vi "2025_day2 - Validate Number.vi"(2 "Number to test In":u64) -> (4 "Reptetive Pattern Found? (Task 2)":bool, 7 "Number to test Out":u64, 8 "Reptetive Pattern Found? (Task 1)":bool)   [LabVIEW 2025]
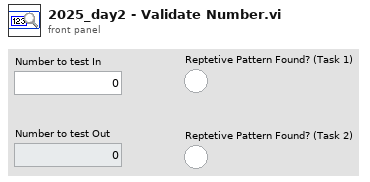
[diagram p1: front panel]
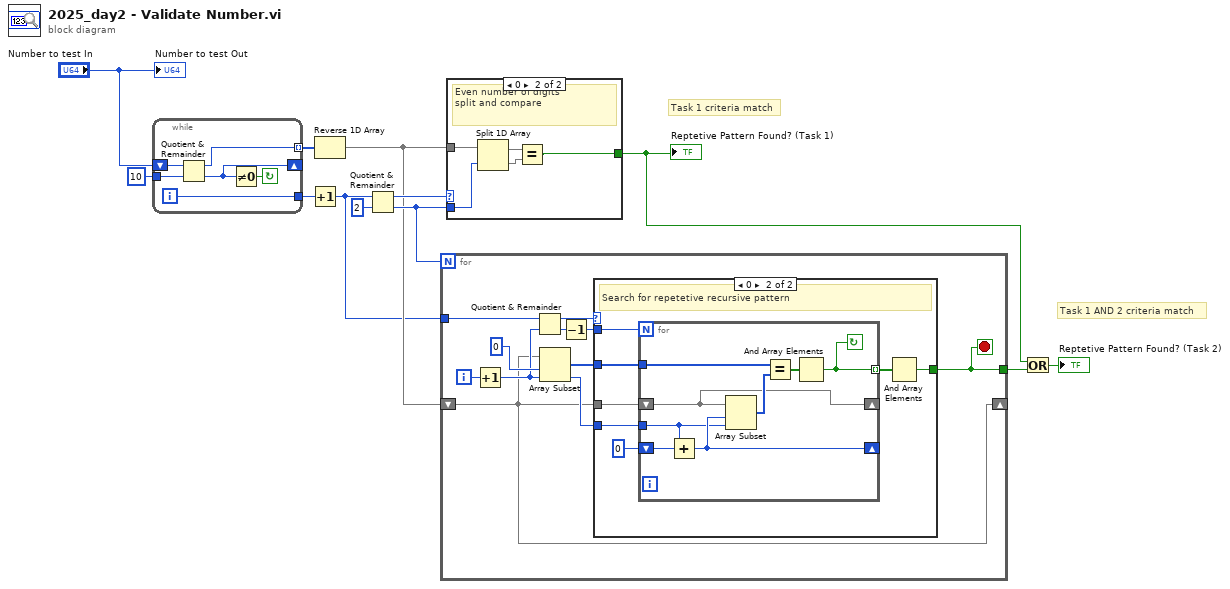
[diagram p0: block diagram]
diagram:
  # "Task 1 AND 2 criteria match"
  # "Task 1 criteria match"
  n1 = while {
    shift-right: [w14] -> _
    shift-left: "Number to test In" -> [w18]
    tunnel: 10 -> [w17]
    tunnel: [w16] -> w11 mode=indexing
    tunnel: [w13] -> w10
    i -> [w13]
    stop <- w15 continue-if-true
    n2 = Quotient & Remainder(x=w18, y=w17) -> (x-y*floor(x/y)=w16:u64, floor(x/y)=w14:u64)
    n3 = Not Equal To 0?(x=w14) -> (x != 0?=w15:bool)
  }
  n4 = Increment(x=w10) -> (x+1=w4:i32)
  n5 = Reverse 1D Array(array=w11) -> (reversed array=w5:u64[])
  n6 = Quotient & Remainder(x=w4, y=2) -> (x-y*floor(x/y)=w8:i32, floor(x/y)=w6:i32)
  n7 = for {
    N: w6 -> [_]
    shift-right: [w21] -> _
    shift-left: w5 -> [w21]
    tunnel: w4 -> [w26]
    tunnel: [w20] -> w3
    i -> [w28]
    stop <- w20 stop-if-true
    n8 = Increment(x=w28) -> (x+1=w23:i32)
    n9 = Quotient & Remainder(x=w26, y=w23) -> (x-y*floor(x/y)=w25:i32, floor(x/y)=w24:i32)
    n10 = Array Subset(array=w21, index=0, length=w23) -> (w22:u64[])
    n11 = Decrement(x=w24) -> (x-1=w19:i32)
    n12 = case shown="0" w25 {
      tunnel: w21 -> [_ w35]
      tunnel: w19 -> [_ w34]
      tunnel: w23 -> [_ w32]
      tunnel: w22 -> [_ w31]
      tunnel: [_ w29] -> w20
      frame Default {
        # "No Match possible"
      }
      frame 0 {
        # "Search for repetetive recursive pattern"
        n13 = for {
          N: w34 -> [_]
          shift-right: [w42] -> _
          shift-left: 0 ("index") -> [w43]
          tunnel: w32 -> [w41]
          tunnel: w31 -> [w40]
          tunnel: [w36] -> w30 mode=indexing
          shift-right: [w37] -> _
          shift-left: w35 -> [w37]
          stop <- w36 continue-if-true
          n14 = Add(x=w43, y=w41) -> (x+y=w42:i32)
          n15 = Array Subset(array=w37, index=w42, length=w41) -> (w39:u64[])
          n16 = Equal?(x=w40, y=w39) -> (x = y?=w38:bool[])
          n17 = And Array Elements(Boolean array=w38) -> (logical AND=w36:bool)
        }
        n18 = And Array Elements(Boolean array=w30) -> (logical AND=w29:bool)
      }
    }
  }
  n19 = case shown="0" w8 {
    tunnel: w6 -> [_ w47]
    tunnel: w5 -> [_ w48]
    tunnel: [_ w44] -> w1
    frame Default {
      # "Odd number of digits"
    }
    frame 0 {
      # "Even number of digits\nsplit and compare"
      n20 = Split 1D Array(array=w48, index=w47) -> (first subarray=w46:u64[], second subarray=w45:u64[])
      n21 = Equal?(x=w46, y=w45) -> (x = y?=w44:bool)
    }
  }
  "Reptetive Pattern Found? (Task 1)" <- w1
  n22 = Or(x=w1, y=w3) -> (x .or. y?=→"Reptetive Pattern Found? (Task 2)":bool)
  "Number to test Out" <- "Number to test In"
